vi "variant2Attributes.vi"(0 "HGF_DIMCommand":refnum<class "HGF_DIMCommand.lvclass">, 2 "rawData":variant, 3 "typeDescriptor":string, 5 "error in (no error)":errorcluster) -> (14 "HGF_DIMCommand":refnum<class "HGF_DIMCommand.lvclass">, 15 "no link":bool, 16 "Parameter":variant, 17 "typeDescriptor":string, 19 "error out":errorcluster)   [LabVIEW 2012, in "HGF_DIM.lvlib" / "HGF_DIMCommand.lvclass"]
doc: "Convert raw data value of variant to variant attributes Pn, n=0,1,2,..."
uses:
  HGF_DIMCommand.lvclass
  HGF_BaseClasses/HGF_PVSubscriber/HGF_PVSubscriber.lvclass
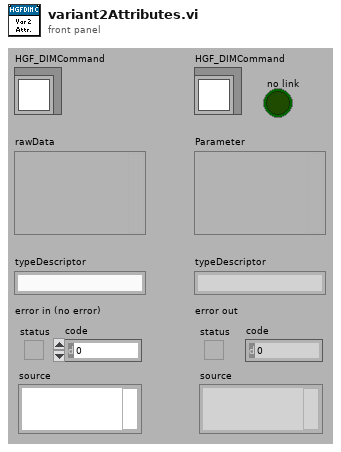
[diagram p1: front panel]
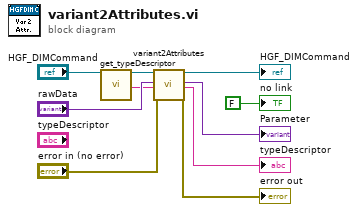
[diagram p0: block diagram]
diagram:
  n1 = call "get_typeDescriptor.vi"("HGF_DIMCommand"="HGF_DIMCommand") -> ("dup HGF_DIMCommand"=w3:refnum<class "HGF_DIMCommand.lvclass">, "typeDescriptor"=w2:string)  [unwired: 1 in, 16 out]
  n2 = call-parent "variant2Attributes.vi"("HGV_PVBase"=w3, "rawData"="rawData", "typeDescriptor"=w2, "error in (no error)"="error in (no error)") -> ("HGV_PVBase"=→"HGF_DIMCommand":refnum<class "HGF_DIMCommand.lvclass">, "Parameter"=→"Parameter":variant, "typeDescriptor"=→"typeDescriptor":string, "error out"=→"error out":errorcluster)  [unwired: 12 out]
  "no link" <- FALSE ("no link")
